vi "DerotatorControl_byYaw2.vi"() -> ()   [LabVIEW 2020]
uses:
  <vilib>/DAQmx/write.llb/DAQmx Write (Digital Bool 1Line 1Point).vi
  <vilib>/DAQmx/create/channels.llb/DAQmx Create Channel (DO-Digital Output).vi
  <vilib>/DAQmx/miscellaneous.llb/DAQmx Fill In Error Info.vi
  GlobalYAW.vi
panel:
  in  "step":bool
  in  "stop":bool
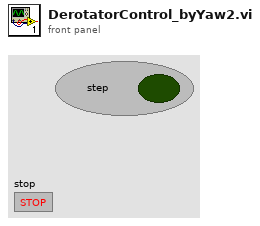
[diagram p1: front panel]
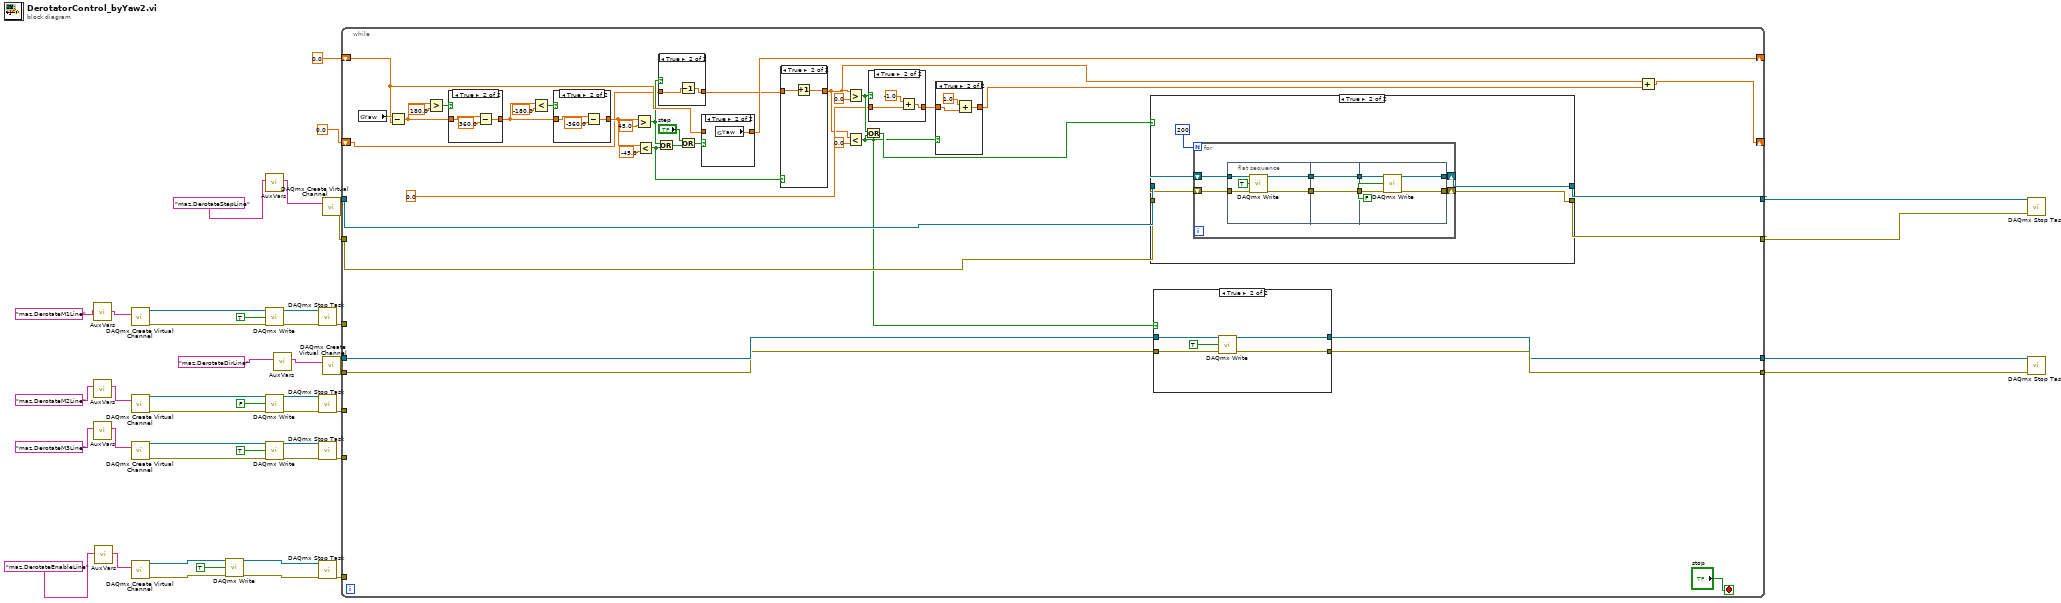
[diagram p0: block diagram]
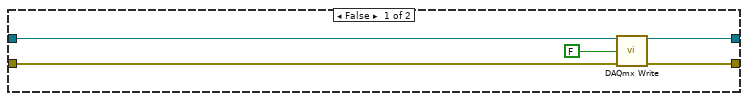
[diagram p9: hidden frame]
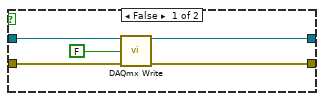
[diagram p10: hidden frame]
diagram:
  n1 = call "AuxVars.vi"("key"="maz.DerotateM1Line") -> ("value"=w13:string)  [unwired: 9 in, 1 out]
  n2 = call "AuxVars.vi"("key"="maz.DerotateM2Line") -> ("value"=w7:string)  [unwired: 9 in, 1 out]
  n3 = call "AuxVars.vi"("key"="maz.DerotateM3Line") -> ("value"=w5:string)  [unwired: 9 in, 1 out]
  n4 = call "AuxVars.vi"("key"="maz.DerotateEnableLine") -> ("value"=w3:string)  [unwired: 9 in, 1 out]
  n5 = call-poly <vilib>:"DAQmx Create Virtual Channel.vi"("lines"=w13) -> ("task out"=w32:refnum<k21>, "error out"=w29:errorcluster)  [unwired: 13 in]
  n6 = call-poly <vilib>:"DAQmx Create Virtual Channel.vi"("lines"=w7) -> ("task out"=w27:refnum<k21>, "error out"=w24:errorcluster)  [unwired: 13 in]
  n7 = call-poly <vilib>:"DAQmx Create Virtual Channel.vi"("lines"=w5) -> ("task out"=w22:refnum<k21>, "error out"=w19:errorcluster)  [unwired: 13 in]
  n8 = call-poly <vilib>:"DAQmx Create Virtual Channel.vi"("lines"=w3) -> ("task out"=w37:refnum<k21>, "error out"=w34:errorcluster)  [unwired: 13 in]
  n9 = call-poly <vilib>:"DAQmx Write.vi"("task/channels in"=w37, "data"=TRUE, "error in"=w34) -> ("task out"=w36:refnum<k21>, "error out"=w35:errorcluster)  [unwired: 10 in, 1 out]
  n10 = call "AuxVars.vi"("key"="maz.DerotateStepLine") -> ("value"=w11:string)  [unwired: 9 in, 1 out]
  n11 = call-poly <vilib>:"DAQmx Write.vi"("task/channels in"=w32, "data"=TRUE, "error in"=w29) -> ("task out"=w31:refnum<k21>, "error out"=w30:errorcluster)  [unwired: 10 in, 1 out]
  n12 = call-poly <vilib>:"DAQmx Write.vi"("task/channels in"=w27, "data"=FALSE, "error in"=w24) -> ("task out"=w26:refnum<k21>, "error out"=w25:errorcluster)  [unwired: 10 in, 1 out]
  n13 = call-poly <vilib>:"DAQmx Write.vi"("task/channels in"=w22, "data"=TRUE, "error in"=w19) -> ("task out"=w21:refnum<k21>, "error out"=w20:errorcluster)  [unwired: 10 in, 1 out]
  n14 = call "AuxVars.vi"("key"="maz.DerotateDirLine") -> ("value"=w9:string)  [unwired: 9 in, 1 out]
  n15 = call <vilib>:"DAQmx Stop Task.vi"("task/channels in"=w31, "error in"=w30) -> ("error out"=w17:errorcluster)  [unwired: 12 in, 1 out]
  n16 = call <vilib>:"DAQmx Stop Task.vi"("task/channels in"=w26, "error in"=w25) -> ("error out"=w16:errorcluster)  [unwired: 12 in, 1 out]
  n17 = call <vilib>:"DAQmx Stop Task.vi"("task/channels in"=w21, "error in"=w20) -> ("error out"=w15:errorcluster)  [unwired: 12 in, 1 out]
  n18 = call <vilib>:"DAQmx Stop Task.vi"("task/channels in"=w36, "error in"=w35) -> ("error out"=w18:errorcluster)  [unwired: 12 in, 1 out]
  n19 = call-poly <vilib>:"DAQmx Create Virtual Channel.vi"("lines"=w11) -> ("task out"=w46:refnum<k21>, "error out"=w45:errorcluster)  [unwired: 13 in]
  n20 = call-poly <vilib>:"DAQmx Create Virtual Channel.vi"("lines"=w9) -> ("task out"=w42:refnum<k21>, "error out"=w41:errorcluster)  [unwired: 13 in]
  n21 = while {
    tunnel: w46 -> [w83]
    tunnel: w45 -> [w82]
    tunnel: [w81] -> w44
    tunnel: [w80] -> w43
    tunnel: w42 -> [w79]
    tunnel: w41 -> [w78]
    tunnel: [w77] -> w40
    tunnel: [w76] -> w39
    tunnel: w18 -> [_]
    tunnel: w17 -> [_]
    tunnel: w16 -> [_]
    tunnel: w15 -> [_]
    shift-right: [w63] -> _
    shift-left: 0.0 ("Yaw") -> [w62]
    shift-right: [w47] -> _
    shift-left: 0.0 ("Yaw") -> [w54]
    stop <- "stop" stop-if-true
    n22 = global read "GlobalYAW.vi" "Yaw"() -> (w75:dbl)
    n23 = Subtract(x=w75, y=w62) -> (x-y=w69:dbl)
    n24 = Greater?(x=w69, y=180.0) -> (0:w68:bool)
    n25 = case shown="True" w68 {
      tunnel: w69 -> [w105 w108]
      tunnel: [w105 w106] -> w64
      frame False {
      }
      frame True {
        n26 = Subtract(x=w108, y=360.0) -> (x-y=w106:dbl)
      }
    }
    n27 = Less?(x=w64, y=-180.0) -> (x < y?=w65:bool)
    n28 = case shown="True" w65 {
      tunnel: w64 -> [w101 w104]
      tunnel: [w101 w102] -> w66
      frame False {
      }
      frame True {
        n29 = Subtract(x=w104, y=-360.0) -> (x-y=w102:dbl)
      }
    }
    n30 = Greater?(x=w66, y=45.0) -> (0:w56:bool)
    n31 = Less?(x=w66, y=-45.0) -> (x < y?=w55:bool)
    n32 = Or(x=w56, y=w55) -> (x .or. y?=w74:bool)
    n33 = case shown="True" w56 {
      tunnel: w54 -> [w93 w94]
      tunnel: [w93 w95] -> w61
      frame False {
      }
      frame True {
        n34 = Decrement(x=w94) -> (x-1=w95:dbl)
      }
    }
    n35 = Or(x="step", y=w74) -> (x .or. y?=w58:bool)
    n36 = case shown="True" w58 {
      tunnel: [w99 w100] -> w63
      tunnel: w62 -> [w99 _]
      frame False {
      }
      frame True {
        n37 = global read "GlobalYAW.vi" "Yaw"() -> (w100:dbl)
      }
    }
    n38 = case shown="True" w55 {
      tunnel: w61 -> [w96 w97]
      tunnel: [w96 w98] -> w48
      frame False {
      }
      frame True {
        n39 = Increment(x=w97) -> (x+1=w98:dbl)
      }
    }
    n40 = Greater?(x=w48, y=0.0) -> (0:w52:bool)
    n41 = Less?(x=w48, y=0.0) -> (x < y?=w51:bool)
    n42 = Or(x=w52, y=w51) -> (x .or. y?=w57:bool)
    n43 = case shown="True" w52 {
      tunnel: 0.0 ("Yaw") -> [w89 w92]
      tunnel: [w89 w91] -> w53
      frame False {
      }
      frame True {
        n44 = Add(x=-1.0, y=w92) -> (x+y=w91:dbl)
      }
    }
    n45 = case shown="True" w51 {
      tunnel: w53 -> [w85 w88]
      tunnel: [w85 w87] -> w49
      frame False {
      }
      frame True {
        n46 = Add(x=1.0, y=w88) -> (x+y=w87:dbl)
      }
    }
    n47 = case shown="True" w57 {
      tunnel: w83 -> [w112 w118]
      tunnel: w82 -> [w111 w117]
      tunnel: [w110 w115] -> w80
      tunnel: [w109 w116] -> w81
      frame False {
        n48 = call-poly <vilib>:"DAQmx Write.vi"("task/channels in"=w112, "data"=FALSE, "error in"=w111) -> ("task out"=w110:refnum<k21>, "error out"=w109:errorcluster)  [unwired: 10 in, 1 out]
      }
      frame True {
        n49 = for {
          N: 200 -> [_]
          shift-right: [w119] -> w115
          shift-left: w118 -> [w122]
          shift-right: [w120] -> w116
          shift-left: w117 -> [w121]
          n50 = flat-sequence {
            tunnel: w122 -> [w130]
            tunnel: w121 -> [w129]
            tunnel: [w128] -> w126
            tunnel: [w127] -> w125
            tunnel: w126 -> [w133]
            tunnel: [w133] -> w124
            tunnel: w125 -> [w132]
            tunnel: [w132] -> w123
            tunnel: [w137] -> w119
            tunnel: [w135] -> w120
            tunnel: w124 -> [w136]
            tunnel: w123 -> [w138]
            frame #0 {
              n51 = call-poly <vilib>:"DAQmx Write.vi"("task/channels in"=w130, "data"=TRUE, "error in"=w129) -> ("task out"=w127:refnum<k21>, "error out"=w128:errorcluster)  [unwired: 10 in, 1 out]
            }
            frame #1 {
            }
            frame #2 {
              n52 = call-poly <vilib>:"DAQmx Write.vi"("task/channels in"=w138, "data"=FALSE, "error in"=w136) -> ("task out"=w137:refnum<k21>, "error out"=w135:errorcluster)  [unwired: 10 in, 1 out]
            }
          }
        }
      }
    }
    n53 = case shown="True" w51 {
      tunnel: w79 -> [w142 w148]
      tunnel: w78 -> [w141 w147]
      tunnel: [w140 w146] -> w76
      tunnel: [w139 w145] -> w77
      frame False {
        n54 = call-poly <vilib>:"DAQmx Write.vi"("task/channels in"=w142, "data"=FALSE, "error in"=w141) -> ("task out"=w140:refnum<k21>, "error out"=w139:errorcluster)  [unwired: 10 in, 1 out]
      }
      frame True {
        n55 = call-poly <vilib>:"DAQmx Write.vi"("task/channels in"=w148, "data"=TRUE, "error in"=w147) -> ("task out"=w146:refnum<k21>, "error out"=w145:errorcluster)  [unwired: 10 in, 1 out]
      }
    }
    n56 = Add(x=w48, y=w49) -> (x+y=w47:dbl)
  }
  n57 = call <vilib>:"DAQmx Stop Task.vi"("task/channels in"=w43, "error in"=w44) -> ()  [unwired: 12 in, 2 out]
  n58 = call <vilib>:"DAQmx Stop Task.vi"("task/channels in"=w39, "error in"=w40) -> ()  [unwired: 12 in, 2 out]
